vi "ParseMsgDigitalIO.vi"(8 "error in":errorcluster, 11 "Sysex Message":u8[](array[numeric]) format="%x") -> (0 "error out":errorcluster, 2 "PortValue":u16, 3 "Port Index":u8, 4 "PortValueAsArray":bool[](array[boolean]))   [LabVIEW 2020, in "FirmataClient.lvlib"]
doc: "Parse a message according to the Firmata Protocol Requirements. \n- https://github.com/firmata/protocol\n- https://github.com/firmata/protocol/blob/master/protocol.md"
uses:
  FirmataClient.lvlib
  controls/FirmataProtocolConstants.ctl
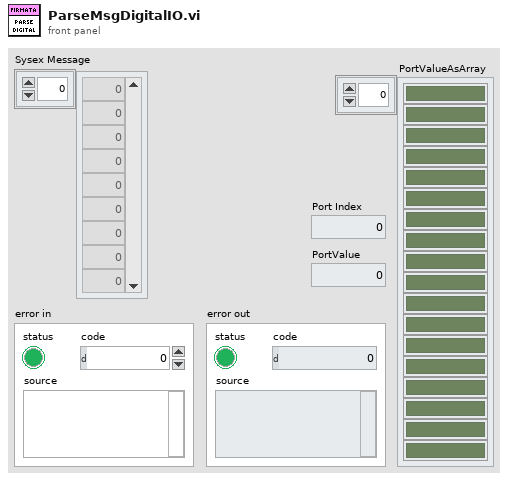
[diagram p1: front panel]
types:
  T1 = typedef "FirmataClient.lvlib/FirmataProtocolConstants.ctl" = u16
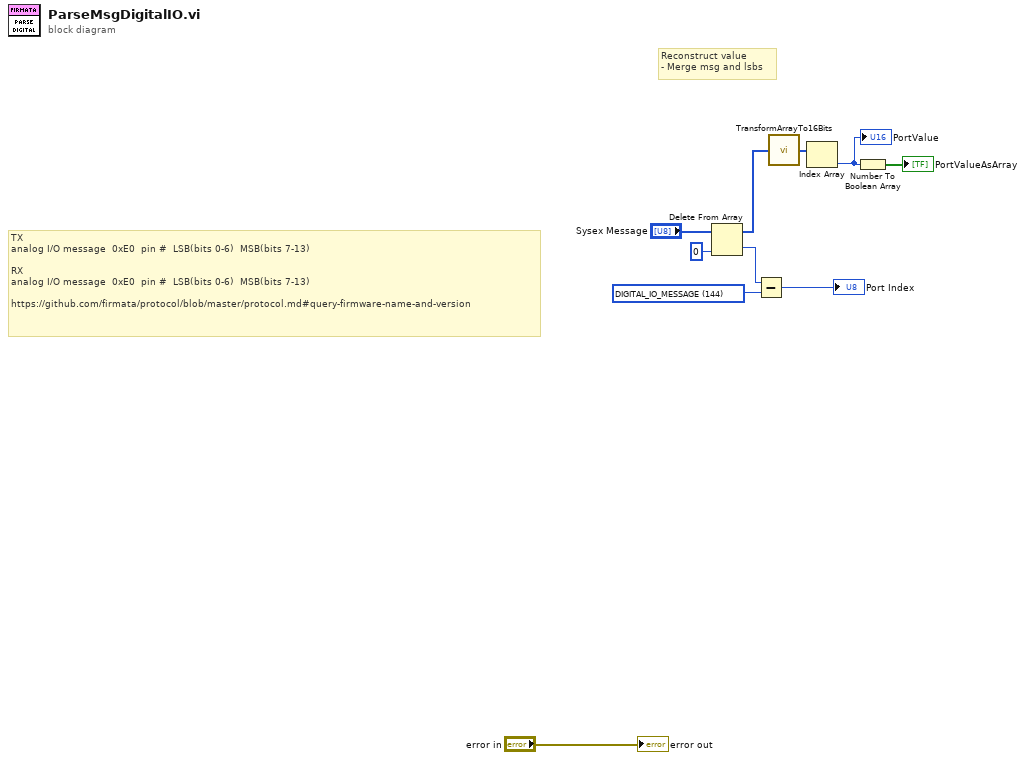
[diagram p0: block diagram]
diagram:
  w7 = T1 144 items=["ANALOG_IO_MESSAGE"=224, "DIGITAL_IO_MESSAGE"=144, "REPORT_ANALOG_PIN"=192, "REPORT_DIGITAL_PORT"=208, "START_SYSEX"=240, "END_SYSEX"=247, "SET_PIN_MODE"=244, "SET_DIGITAL_PIN_VALUE"=245, "PROTOCOL_VERSION"=249, "SYSTEM_RESET"=255, "SYSEX.EXTENDED_ID"=0, "SYSEX.RESERVED_USER_COMMANDs"=1, "SYSEX.ANALOG_MAPPING_QUERY"=105, "SYSEX.ANALOG_MAPPING_RESPONSE"=106, "SYSEX.CAPABILITY_QUERY"=107, "SYSEX.CAPABILITY_RESPONSE"=108, "SYSEX.PIN_STATE_QUERY"=109, "SYSEX.PIN_STATE_RESPONSE"=110, "SYSEX.REPORT_FIRMWARE"=121, "SYSEX.EXTENDED_ANALOG"=111, "SYSEX.STRING_DATA"=113, "SYSEX.REALTIME"=127, "SYSEX.NON_REALTIME"=126, "SYSEX.SAMPLING_INTERVAL"=122] ("FimataProtocolConstants")
  # "Reconstruct value\n- Merge msg and lsbs"
  # "TX\nanalog I/O message \t0xE0 \tpin # \tLSB(bits 0-6) \tMSB(bits 7-13)\n\nRX\nanalog I/O message \t0xE0 \tpin # \tLSB(bits 0-6) \tMSB(bits 7-13)\n\nhttps://github.com/firmata/protocol/blob/master/protocol.md#query-firmware-name-and-version"
  n1 = Delete From Array(array="Sysex Message", index=0) -> (deleted portion=w4:u8, array with subset deleted=w3:u8[])  [unwired: 1 in]
  n2 = Subtract(x=w4, y=w7) -> (x-y=→"Port Index":T1)
  n3 = call "TransformArrayTo16Bits.vi"("Bytes In"=w3) -> ("Byte Out"=w2:u16[])
  n4 = Index Array(array=w2) -> (element=w1:u16)  [unwired: 1 in]
  "PortValue" <- w1
  n5 = Number To Boolean Array(number=w1) -> (Boolean array=→"PortValueAsArray":bool[])
  "error out" <- "error in"
